vi "Remove Quotes from String if Present.vi"(11 "String":string) -> (3 "String with Quotes Removed":string)   [LabVIEW 2020, in "JKI State Machine API.lvlib" / "JKI SM.lvclass"]
uses:
  JKI SM.lvclass
  JKI SM.lvclass/JKI SM.ctl
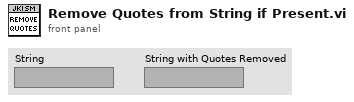
[diagram p1: front panel]
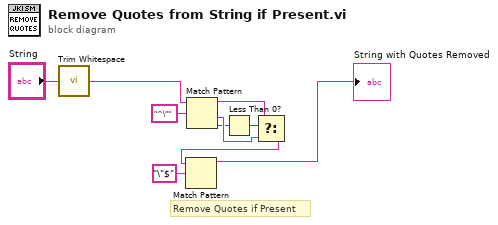
[diagram p0: block diagram]
diagram:
  # "Remove Quotes if Present"
  n1 = call <vilib>:"Trim Whitespace.vi"("string"="String") -> ("trimmed string"=w1:string)  [unwired: 1 in]
  n2 = Match Pattern(string=w1, regular expression="^\"") -> (before substring=w6:string, after substring=w7:string, offset past match=w4:i32)  [unwired: 1 in, 1 out]
  n3 = Less Than 0?(x=w4) -> (x < 0?=w5:bool)
  n4 = Select(t=w6, s=w5, f=w7) -> (s? t:f=w10:string)
  n5 = Match Pattern(string=w10, regular expression="\"$") -> (before substring=→"String with Quotes Removed":string)  [unwired: 1 in, 3 out]
